vi "GetClusterValueRec.vi"(0 "Controls[] In":refnum<vi>[](array[refnum]), 7 "Array":string[](array[string]), 11 "error in (no error)":errorcluster) -> (4 "Controls[] Out":refnum<vi>[](array[refnum]), 8 "Control Value":variant, 15 "error out":errorcluster)   [LabVIEW 2016]
doc: "This VI gets value for the controls present n other VI"
uses:
  <vilib>/ErrorRing/Error Ring.xnode
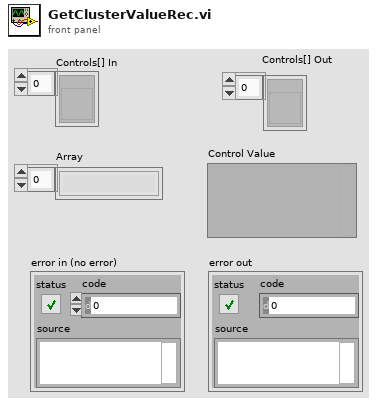
[diagram p1: front panel]
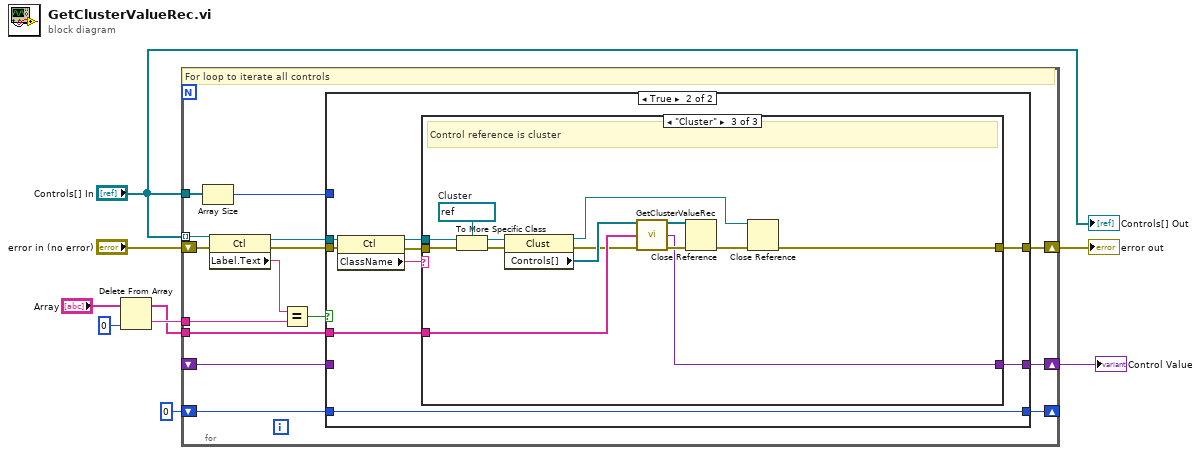
[diagram p0: block diagram]
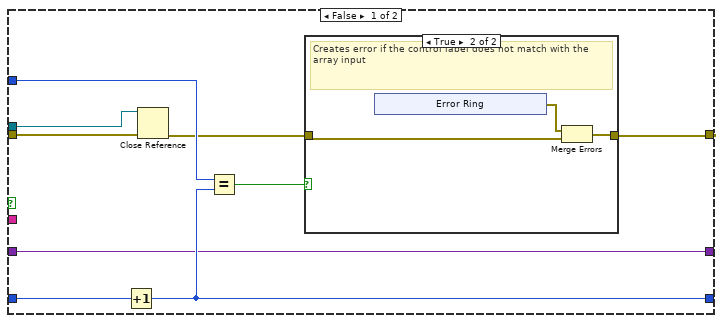
[diagram p2: hidden frame]
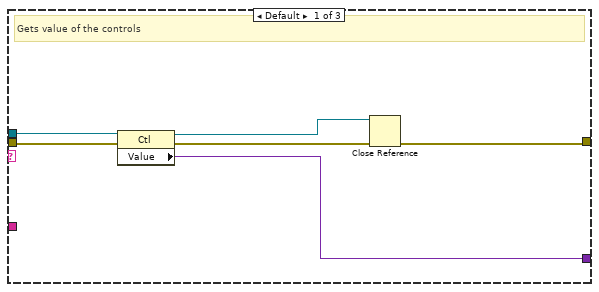
[diagram p4: hidden frame]
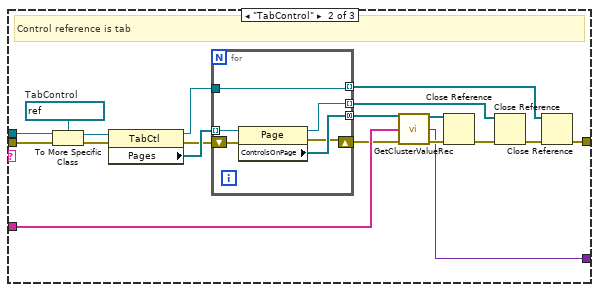
[diagram p5: hidden frame]
diagram:
  n1 = Delete From Array(array="Array", index=0) -> (deleted portion=w7:string, array with subset deleted=w6:string[])  [unwired: 1 in]
  n2 = for {
    tunnel: "Controls[] In" -> [w24] mode=indexing
    tunnel: w7 -> [w21]
    tunnel: w6 -> [w19]
    shift-right: [w16] -> w3
    shift-left: "error in (no error)" -> [w18]
    tunnel: "Controls[] In" -> [w15]
    shift-right: [w12] -> _
    shift-left: 0 -> [w13]
    shift-right: [w11] -> w1
    shift-left: _ -> [w10]
    # "For loop to iterate all controls"
    n3 = Array Size(array=w15) -> (size(s)=w14:i32)
    n4 = property class="Ctl"(reference=w24, error in=w18) -> (reference out=w20:refnum<vi>, error out=w17:errorcluster, "Label.Text"=w22:string)
    n5 = Equal?(x=w22, y=w21) -> (x = y?=w23:bool)
    n6 = case shown="True" w23 {
      tunnel: w20 -> [w33 w47]
      tunnel: w19 -> [_ w45]
      tunnel: w17 -> [w32 w44]
      tunnel: [w27 w42] -> w16
      tunnel: w14 -> [w29 _]
      tunnel: w13 -> [w31 w41]
      tunnel: [w30 w41] -> w12
      tunnel: [w25 w39] -> w11
      tunnel: w10 -> [w25 _]
      frame False {
        n7 = Increment(x=w31) -> (x+1=w30:i32)
        n8 = Close Reference(reference=w33, error in (no error)=w32) -> (error out=w26:errorcluster)
        n9 = Equal?(x=w29, y=w30) -> (x = y?=w28:bool)
        n10 = case shown="True" w28 {
          tunnel: [w34 w37] -> w27
          tunnel: w26 -> [w34 w35]
          frame False {
            # "Does not create error if the control label matchs with the array input"
          }
          frame True {
            # "Creates error if the control label does not match with the array input"
            n11 = xnode "Error Ring"() -> ("error out"=w36:errorcluster)
            n12 = Merge Errors(w36, w35) -> (w37:errorcluster)
          }
        }
      }
      frame True {
        n13 = property class="Ctl"(reference=w47, error in=w44) -> (reference out=w40:refnum<vi>, error out=w43:errorcluster, "ClassName"=w46:string)
        n14 = case shown="\"Cluster\"" w46 {
          tunnel: w40 -> [w53 w69 w92]
          tunnel: w45 -> [_ w58 w83]
          tunnel: w43 -> [w52 w67 w88]
          tunnel: [w50 w62 w86] -> w42
          tunnel: [w48 w55 w79] -> w39
          frame Default {
            # "Gets value of the controls"
            n15 = property class="Ctl"(reference=w53, error in=w52) -> (reference out=w49:refnum<vi>, error out=w51:errorcluster, "Value"=w48:variant)
            n16 = Close Reference(reference=w49, error in (no error)=w51) -> (error out=w50:errorcluster)
          }
          frame "TabControl" {
            w72 = refnum<vi> refnum  # TabControl
            # "Control reference is tab"
            n17 = To More Specific Class(target class=w72, reference=w69, error in=w67) -> (specific class reference=w71:refnum<vi>, error out=w70:errorcluster)
            n18 = property class="TabCtl"(reference=w71, error in=w70) -> (reference out=w65:refnum<vi>, error out=w66:errorcluster, "Pages"=w68:refnum<vi>[])
            n19 = for {
              tunnel: w68 -> [w78] mode=indexing
              tunnel: [w77] -> w59 mode=concatenating
              shift-right: [w75] -> w57
              shift-left: w66 -> [w76]
              tunnel: [w74] -> w61 mode=indexing
              tunnel: [w73] -> w60 mode=indexing
              tunnel: w65 -> [w73]
              n20 = property class="Page"(reference=w78, error in=w76) -> (reference out=w74:refnum<vi>, error out=w75:errorcluster, "ControlsOnPage"=w77:refnum<vi>[])
            }
            n21 = call "GetClusterValueRec.vi"("Controls[] In"=w59, "Array"=w58, "error in (no error)"=w57) -> ("Controls[] Out"=w54:refnum<vi>[], "Control Value"=w55:variant, "error out"=w56:errorcluster)  [unwired: 10 in]
            n22 = Close Reference(reference=w54, error in (no error)=w56) -> (error out=w64:errorcluster)
            n23 = Close Reference(reference=w61, error in (no error)=w64) -> (error out=w63:errorcluster)
            n24 = Close Reference(reference=w60, error in (no error)=w63) -> (error out=w62:errorcluster)
          }
          frame "Cluster" {
            w91 = refnum<vi> refnum  # Cluster
            # "Control reference is cluster"
            n25 = To More Specific Class(target class=w91, reference=w92, error in=w88) -> (specific class reference=w90:refnum<vi>, error out=w89:errorcluster)
            n26 = property class="Clust"(reference=w90, error in=w89) -> (reference out=w85:refnum<vi>, error out=w82:errorcluster, "Controls[]"=w84:refnum<vi>[])
            n27 = call "GetClusterValueRec.vi"("Controls[] In"=w84, "Array"=w83, "error in (no error)"=w82) -> ("Controls[] Out"=w80:refnum<vi>[], "Control Value"=w79:variant, "error out"=w81:errorcluster)  [unwired: 10 in]
            n28 = Close Reference(reference=w80, error in (no error)=w81) -> (error out=w87:errorcluster)
            n29 = Close Reference(reference=w85, error in (no error)=w87) -> (error out=w86:errorcluster)
          }
        }
      }
    }
  }
  "Control Value" <- w1
  "error out" <- w3
  "Controls[] Out" <- "Controls[] In"
